vi "CLD 12 Sequencer State Machine solution Two.vi"() -> ()   [LabVIEW 2019]
doc: "CLD 12: Sequences boolean values in the order they are loaded from the file."
uses:
  CLD 12 Data Cluster.ctl
  CLD 12 Sequencer Enum.ctl
  CLD3 FGV Mode.ctl
panel:
  out "Current Time Target":dbl
  in  "error in (no error)":errorcluster
  out "error out":errorcluster
  in  "Stop Button":bool
  out "Time Elapsed":dbl
  out "Switch 3":bool
  out "Switch 2":bool
  out "Switch 1":bool
  in  "Start":bool
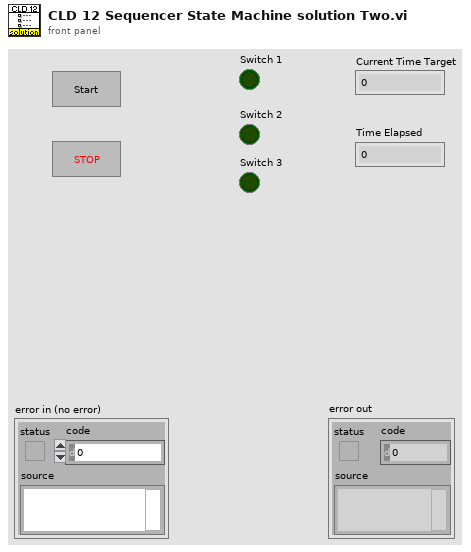
[diagram p1: front panel]
types:
  T1 = typedef "CLD 12 Data Cluster.ctl" = cluster{"Command":T2, "Time Value":dbl, "Boolean":bool, "Boolean 2":bool, "Boolean 3":bool}
  T2 = typedef "CLD 12 Sequencer Enum.ctl" = enum16{"Initialize", "SetTime", "RunState1", "Runstate2", "Idle", "Start"}
  T3 = typedef "CLD3 FGV Mode.ctl" = enum16{"Start Timer", "Reset Timer", "Read Time", "Pause", "Resume"}
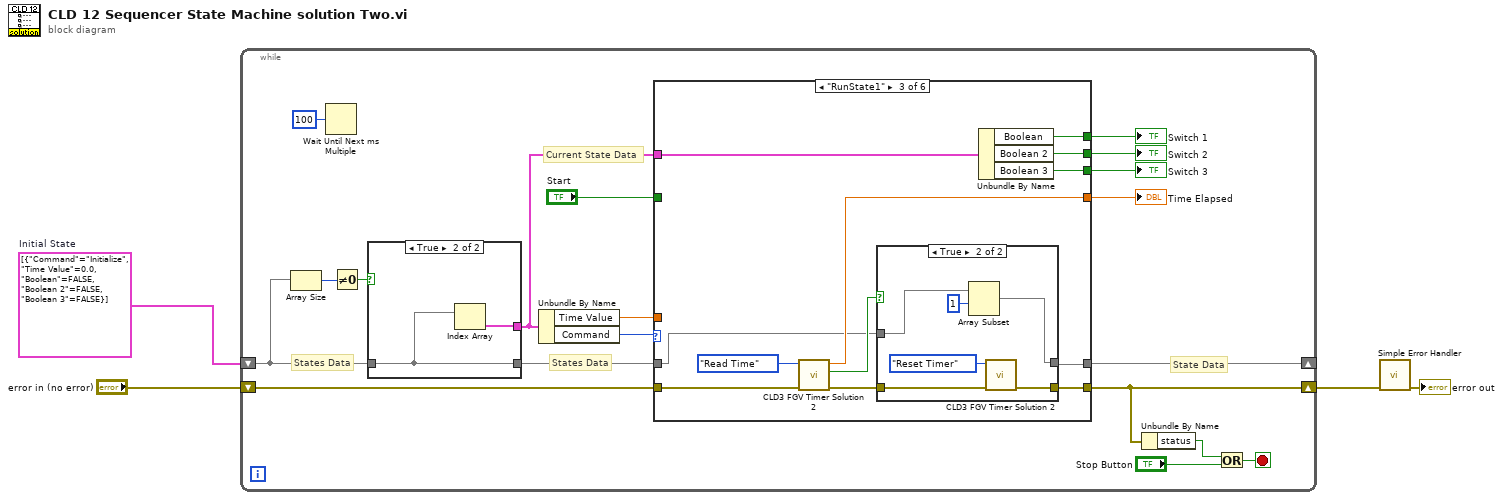
[diagram p0: block diagram]
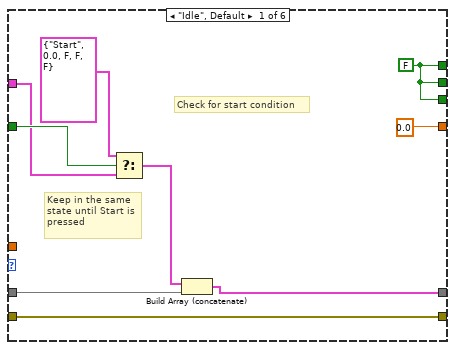
[diagram p2: hidden frame]
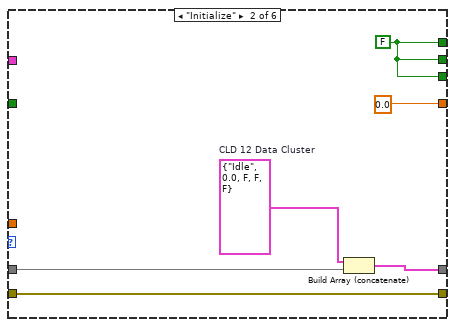
[diagram p3: hidden frame]
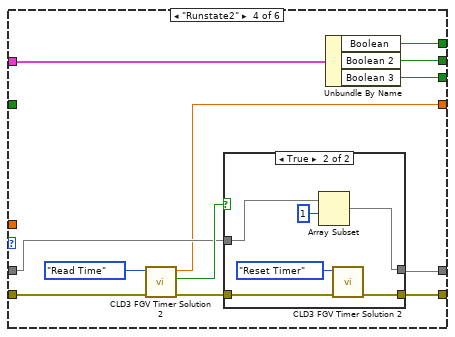
[diagram p5: hidden frame]
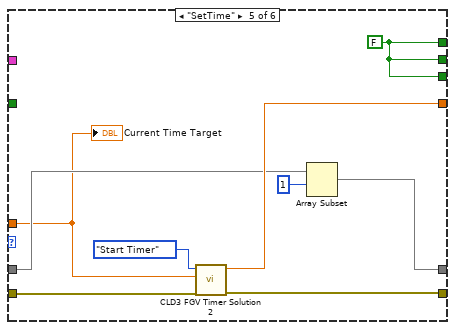
[diagram p7: hidden frame]
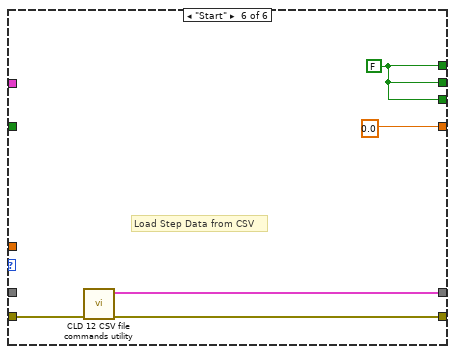
[diagram p8: hidden frame]
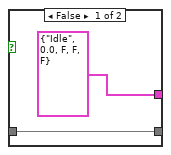
[diagram p9: hidden frame]
diagram:
  w1 = T1[] [{"Command"=enum."Initialize", "Time Value"=0.0, "Boolean"=FALSE, "Boolean 2"=FALSE, "Boolean 3"=FALSE}]  # Initial State
  n1 = while {
    shift-right: [w21] -> w2
    shift-left: "error in (no error)" -> [w19]
    shift-right: [w7] -> _
    shift-left: w1 -> [w11]
    stop <- w22 stop-if-true
    # "Current State Data"
    # "States Data"
    # "State Data"
    # "States Data"
    n2 = Array Size(array=w11) -> (size(s)=w10:i32)
    n3 = Wait Until Next ms Multiple(millisecond multiple=u32 100) -> ()  [unwired: 1 out]
    n4 = Not Equal To 0?(x=w10) -> (x != 0?=w9:bool)
    n5 = case shown="True" w9 {
      tunnel: [T1 {"Command"=enum."Idle", "Time Value"=0.0, "Boolean"=FALSE, "Boolean 2"=FALSE, "Boolean 3"=FALSE} ("CLD 12 Data Cluster") w96] -> w13
      tunnel: w11 -> [w93 w95]
      tunnel: [w93 w95] -> w8
      frame False {
      }
      frame True {
        n6 = Index Array(array=w95) -> (element=w96:T1)  [unwired: 1 in]
      }
    }
    n7 = Unbundle By Name(w13) -> ("Time Value"=w12:dbl, "Command"=w14:T2)
    n8 = case shown="\"RunState1\"" w14 {
      tunnel: [w28 w38 w42 w67 w85 w91] -> w21
      tunnel: w19 -> [w28 w38 w49 w64 w86 w92]
      tunnel: [w32 w37 w47 w61 w87 w90] -> w18
      tunnel: [w32 w37 w46 w60 w87 w90] -> w17
      tunnel: [w32 w37 w45 w59 w87 w90] -> w16
      tunnel: [0.0 ("Elapsed Time (s.ss)") 0.0 ("Elapsed Time (s.ss)") w48 w62 w83 0.0 ("Elapsed Time (s.ss)")] -> w15
      tunnel: [w29 w35 w40 w66 w80 w89] -> w7
      tunnel: w13 -> [w26 _ w39 w63 _ _]
      tunnel: w12 -> [_ _ _ _ w79 _]
      tunnel: w8 -> [w30 w36 w41 w65 w81 _]
      tunnel: "Start" -> [w27 _ _ _ _ _]
      frame "Idle", Default {
        w32 = FALSE ("Boolean 1")
        # "Keep in the same \nstate until Start is \npressed"
        # "Check for start condition"
        n9 = Select(t=T1 {"Command"=enum."Start", "Time Value"=0.0, "Boolean"=FALSE, "Boolean 2"=FALSE, "Boolean 3"=FALSE}, s=w27, f=w26) -> (s? t:f=w25:T1)
        n10 = Build Array (concatenate)(w25, w30) -> (w29:T1[])
      }
      frame "Initialize" {
        w37 = FALSE ("Boolean 1")
        w33 = T1 {"Command"=enum."Idle", "Time Value"=0.0, "Boolean"=FALSE, "Boolean 2"=FALSE, "Boolean 3"=FALSE}  # CLD 12 Data Cluster
        n11 = Build Array (concatenate)(w33, w36) -> (w35:T1[])
      }
      frame "RunState1" {
        n12 = call "CLD3 FGV Timer Solution 2.vi"("Error In"=w49, "Timer Mode"=CLD3_FGV_Mode."Read Time") -> ("Error Out"=w43:errorcluster, "Has Time Elapsed"=w44:bool, "Elapsed Time (s.ss)"=w48:dbl)  [unwired: 7 in]
        n13 = case shown="True" w44 {
          tunnel: w43 -> [w51 w58]
          tunnel: [w51 w57] -> w42
          tunnel: w41 -> [w52 w55]
          tunnel: [w52 w53] -> w40
          frame False {
          }
          frame True {
            n14 = Array Subset(array=w55, index=1) -> (w53:T1[])  [unwired: 1 in]
            n15 = call "CLD3 FGV Timer Solution 2.vi"("Error In"=w58, "Timer Mode"=CLD3_FGV_Mode."Reset Timer") -> ("Error Out"=w57:errorcluster)  [unwired: 7 in, 2 out]
          }
        }
        n16 = Unbundle By Name(w39) -> ("Boolean"=w47:bool, "Boolean 2"=w46:bool, "Boolean 3"=w45:bool)
      }
      frame "Runstate2" {
        n17 = call "CLD3 FGV Timer Solution 2.vi"("Error In"=w64, "Timer Mode"=CLD3_FGV_Mode."Read Time") -> ("Error Out"=w68:errorcluster, "Has Time Elapsed"=w69:bool, "Elapsed Time (s.ss)"=w62:dbl)  [unwired: 7 in]
        n18 = case shown="True" w69 {
          tunnel: w68 -> [w71 w78]
          tunnel: [w71 w77] -> w67
          tunnel: w65 -> [w72 w75]
          tunnel: [w72 w73] -> w66
          frame False {
          }
          frame True {
            n19 = Array Subset(array=w75, index=1) -> (w73:T1[])  [unwired: 1 in]
            n20 = call "CLD3 FGV Timer Solution 2.vi"("Error In"=w78, "Timer Mode"=CLD3_FGV_Mode."Reset Timer") -> ("Error Out"=w77:errorcluster)  [unwired: 7 in, 2 out]
          }
        }
        n21 = Unbundle By Name(w63) -> ("Boolean"=w61:bool, "Boolean 2"=w60:bool, "Boolean 3"=w59:bool)
      }
      frame "SetTime" {
        w87 = FALSE ("Boolean 1")
        n22 = call "CLD3 FGV Timer Solution 2.vi"("Error In"=w86, "Time Target (s)"=w79, "Timer Mode"=CLD3_FGV_Mode."Start Timer") -> ("Error Out"=w85:errorcluster, "Elapsed Time (s.ss)"=w83:dbl)  [unwired: 6 in, 1 out]
        n23 = Array Subset "Array Subset"(array=w81, index=1) -> (w80:T1[])  [unwired: 1 in]
        "Current Time Target" <- w79
      }
      frame "Start" {
        w90 = FALSE ("Boolean 1")
        # "Load Step Data from CSV"
        n24 = call "CLD 12 CSV file commands utility.vi"("Error In"=w92) -> ("Error Out"=w91:errorcluster, "Command Array Out"=w89:T1[])  [unwired: 9 in]
      }
    }
    "Time Elapsed" <- w15
    "Switch 1" <- w18
    "Switch 2" <- w17
    "Switch 3" <- w16
    n25 = Unbundle By Name(w21) -> ("status"=w20:bool)
    n26 = Or(x=w20, y="Stop Button") -> (x .or. y?=w22:bool)
  }
  n27 = call <vilib>:"Simple Error Handler.vi"("error in (no error)"=w2) -> ("error out"=→"error out":errorcluster)  [unwired: 4 in, 4 out]
